vi "曲线模型属性写入.vi"(4 "error in (no error)":errorcluster caption="错误输入（无错误）", 5 "Value":cluster{"参数":u8, "测量模式":u8, "量程":u8} caption="值", 6 "Container State":T2 caption="容器状态", 7 "Display State In":T1 caption="显示状态输入" {"校准时间"."标液校准时间4" format="%<%Y/%m/%d %H:%M:%S>T"; "校准时间"."标液校准时间3" format="%<%Y/%m/%d %H:%M:%S>T"; "校准时间"."标液校准时间2" format="%<%Y/%m/%d %H:%M:%S>T"; "校准时间"."标液校准时间1" format="%<%Y/%m/%d %H:%M:%S>T"; "校准时间"."零点校准时间" format="%<%Y/%m/%d %H:%M:%S>T"}) -> (0 "error out":errorcluster caption="错误输出", 3 "Display State Out":T1 caption="显示状态输出" {"校准时间"."标液校准时间4" format="%<%Y/%m/%d %H:%M:%S>T"; "校准时间"."标液校准时间3" format="%<%Y/%m/%d %H:%M:%S>T"; "校准时间"."标液校准时间2" format="%<%Y/%m/%d %H:%M:%S>T"; "校准时间"."标液校准时间1" format="%<%Y/%m/%d %H:%M:%S>T"; "校准时间"."零点校准时间" format="%<%Y/%m/%d %H:%M:%S>T"})   [LabVIEW 2016, in "曲线模型.xctl"]
uses:
  <vilib>/_xctls/Container State.ctl
  <vilib>/_xctls/XControlSupport.lvlib
panel:
  # "将以下值显示控件替换为所需类型的显示控件。\n不要从连线板中删除该显示控件或其它显示控件。\n不要更改连线板模式。\n值显示控件应始终位于连线板输出端自顶部起第三个接线端。"
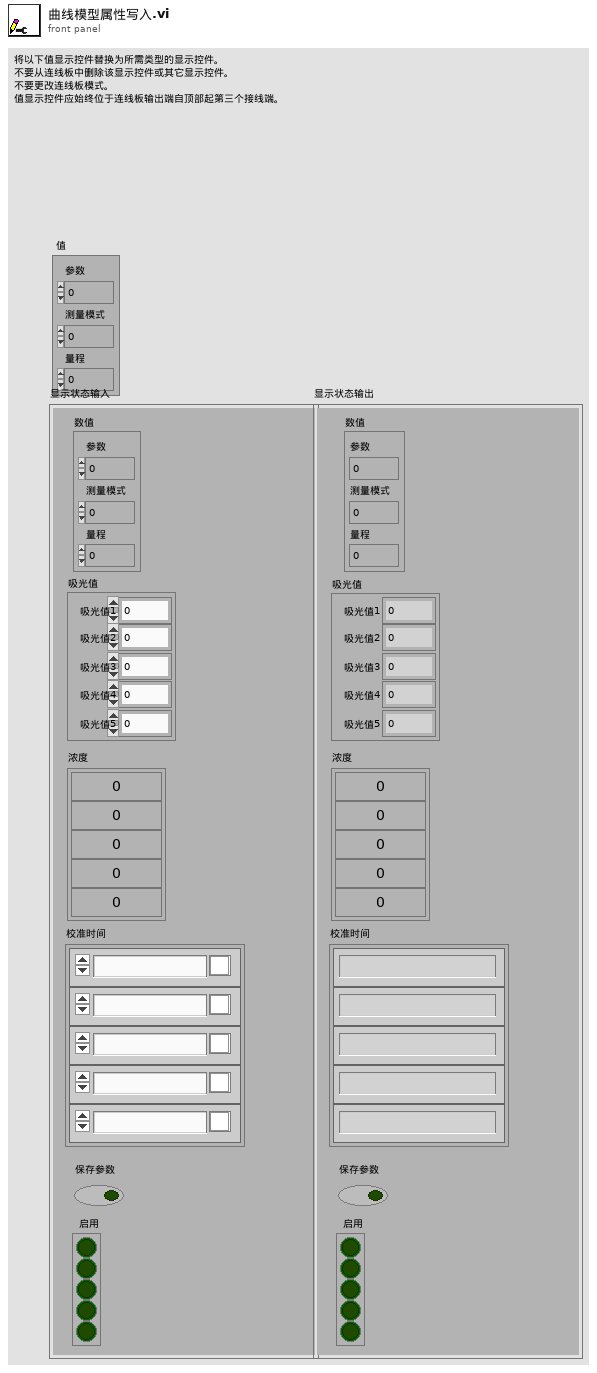
[diagram p1: front panel]
types:
  T1 = typedef "曲线模型.xctl/状态 1.ctl" = cluster{"模型选择":cluster{"参数":u8, "测量模式":u8, "量程":u8}, "吸光值":cluster{"Value":dbl, "Value 2":dbl, "Value 3":dbl, "Value 4":dbl, "Value 5":dbl}, "浓度":cluster{"标液浓度1":dbl, "标液浓度2":dbl, "标液浓度3":dbl, "标液浓度4":dbl, "标液浓度5":dbl}, "校准时间":cluster{"零点校准时间":timestamp, "标液校准时间1":timestamp, "标液校准时间2":timestamp, "标液校准时间3":timestamp, "标液校准时间4":timestamp}, "保存参数":bool, "启用":cluster{"启用":bool, "启用 2":bool, "启用 3":bool, "启用 4":bool, "启用 5":bool}}
  T2 = typedef "XControlSupport.lvlib/Container State.ctl" = cluster{"Indicator?":bool, "Run Mode?":bool, " Refnum":refnum<vi>}
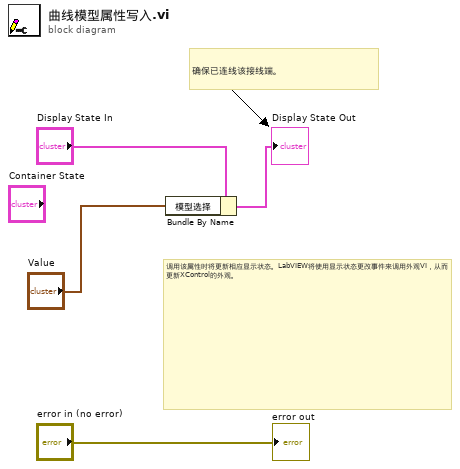
[diagram p0: block diagram]
diagram:
  # "确保已连线该接线端。"
  # "调用该属性时将更新相应显示状态。LabVIEW将使用显示状态更改事件来调用外观VI，从而更新XControl的外观。"
  n1 = Bundle By Name(cluster="Display State In", "模型选择"="Value") -> (→"Display State Out":T1)
  "error out" <- "error in (no error)"
